vi "EventPassState.vi"(10 "IA State Input":T1) -> (1 "Id":dbl, 2 "IA State Output":T1, 3 "Pass State":bool)   [LabVIEW 2017]
uses:
  Core/AI Input.ctl
  Core/AI Robot.ctl
  Intel/Functions Enum.ctl
  Intel/AttackerStates.ctl
  Core/AI Ball.ctl
  Core/Field Size.ctl
  Core/AI Judge.ctl
  Intel/Command Enum.ctl
  Events.ctl
panel:
  in  "Desabilita passe":bool=TRUE
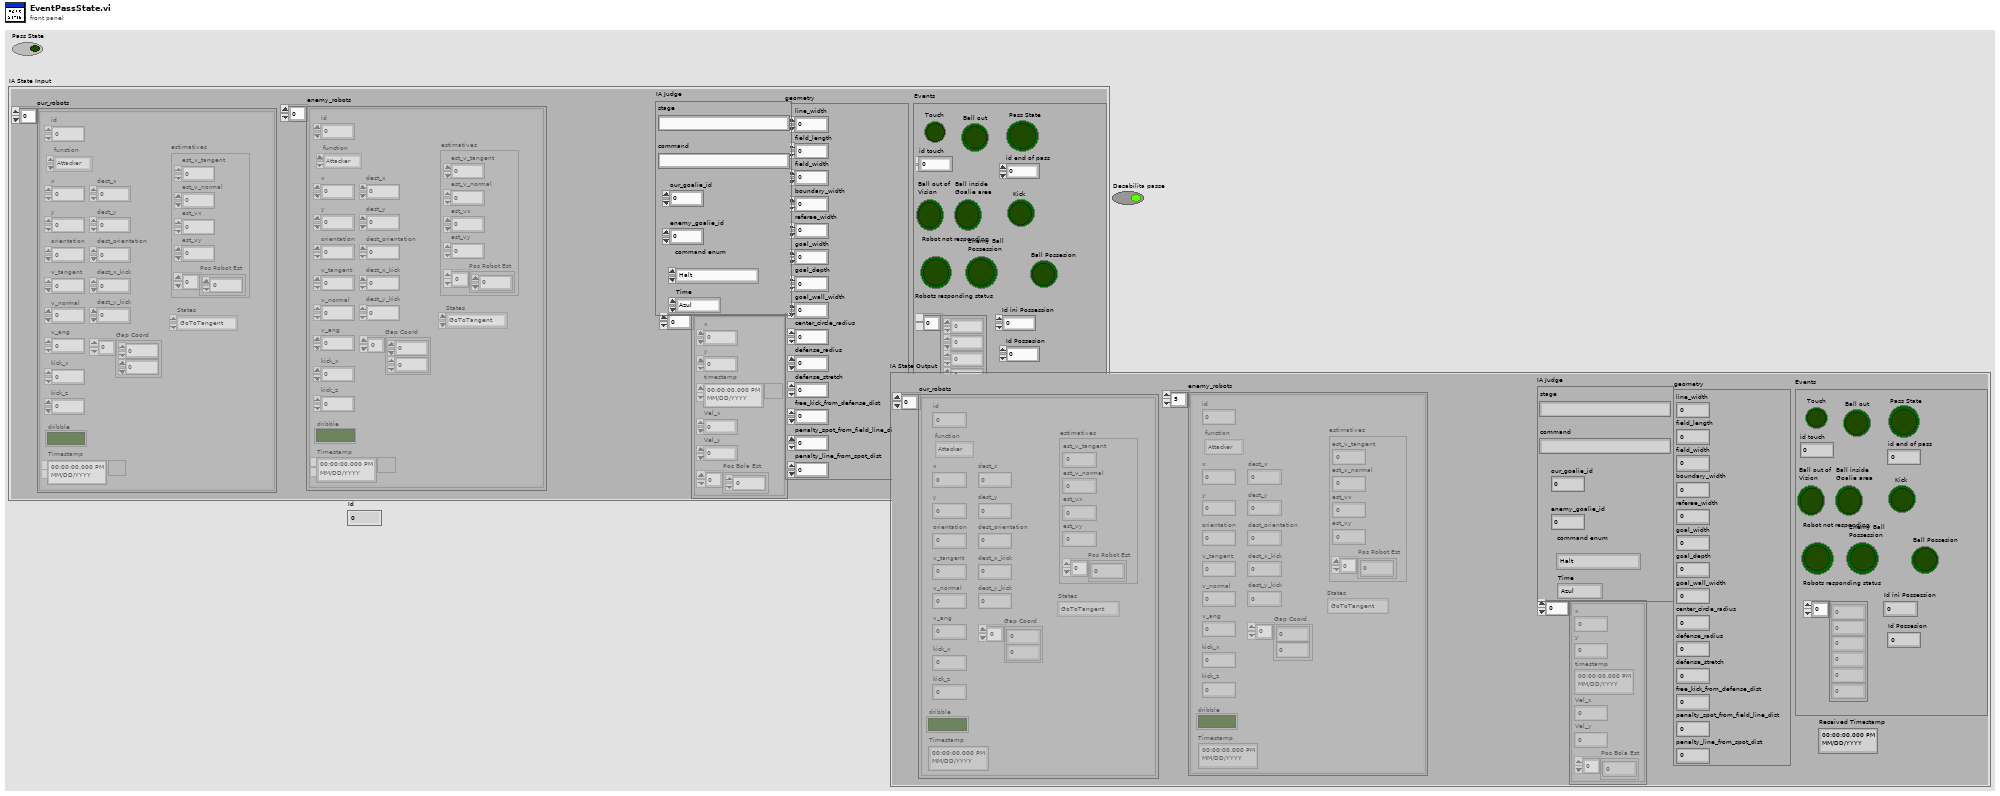
[diagram p1: front panel]
types:
  T1 = typedef "AI Input.ctl" = cluster{"our_robots":T2[], "enemy_robots":T2[], "balls":T5[], "geometry":T6, "IA Judge":T7, "Received Timestamp":timestamp, "Events":T9}
  T2 = typedef "AI Robot.ctl" = cluster{"id":u32, "function":T3, "x":dbl, "y":dbl, "orientation":dbl, "v_tangent":dbl, "v_normal":dbl, "v_ang":dbl, "kick_x":dbl, "kick_z":dbl, "dribble":bool, "Timestamp":timestamp, "dest_x":dbl, "dest_y":dbl, "dest_orientation":dbl, "estimatives":cluster{"est_v_tangent":dbl, "est_v_normal":dbl, "est_vx":dbl, "est_vy":dbl, "Pos Robot Est":dbl[]}, "dest_x_kick":dbl, "dest_y_kick":dbl, "Gap Coord":dbl[], "States":T4}
  T3 = typedef "Functions Enum.ctl" = enum16{"Attacker", "Goalie", "Defender", "Striker", "Goto 0", "Dummy", "Kicker", "ZigZag"}
  T4 = typedef "AttackerStates.ctl" = enum16{"Pass", "GoToTangent", "BallGetting", "GoToKick", ""}
  T5 = typedef "AI Ball.ctl" = cluster{"x":dbl, "y":dbl, "timestamp":timestamp, "Vel_x":dbl, "Vel_y":dbl, "Pos Bola Est":dbl[]}
  T6 = typedef "Field Size.ctl" = cluster{"line_width":u32, "field_length":u32, "field_width":u32, "boundary_width":u32, "referee_width":u32, "goal_width":u32, "goal_depth":u32, "goal_wall_width":u32, "center_circle_radius":u32, "defense_radius":u32, "defense_stretch":u32, "free_kick_from_defense_dist":u32, "penalty_spot_from_field_line_dist":u32, "penalty_line_from_spot_dist":u32}
  T7 = typedef "AI Judge.ctl" = cluster{"stage":string, "command":string, "our_goalie_id":dbl, "enemy_goalie_id":dbl, "command enum":T8, "Time":enum16{"Azul", "Amarelo"}}
  T8 = typedef "Command Enum.ctl" = enum16{"Halt", "Stop", "Force Start", "PKA Normal Start", "Prepare Kickoff Ally", "PKE Normal Start", "Prepare Kickoff Enemy", "Prepare Penalty Ally", "PPA Normal Start", "Prepare Penalty Enemy", "PPE Normal Start", "Direct Free Enemy", "Direct Free Ally", "Indirect Free Enemy", "Indirect Free Ally", "Timeout Enemy", "Timeout Ally", "Goal Enemy", "Goal Ally", "Ball Placement Enemy", "Ball Placement Ally", "Normal Half Time", "Extra Time Break", "Extra Half Time", "None", "Post Game"}
  T9 = typedef "Events.ctl" = cluster{"Touch":bool, "Ball out":bool, "id touch":dbl, "Ball out of \nVision":bool, "Ball inside \nGoalie area":bool, "Robot not responding":bool, "Robots responding status":dbl[], "Enemy Ball \nPossession":bool, "Pass State":bool, "id end of pass":dbl, "Kick":bool, "Id ini Possession":dbl, "Ball Possesion":bool, "Id Possesion":dbl}
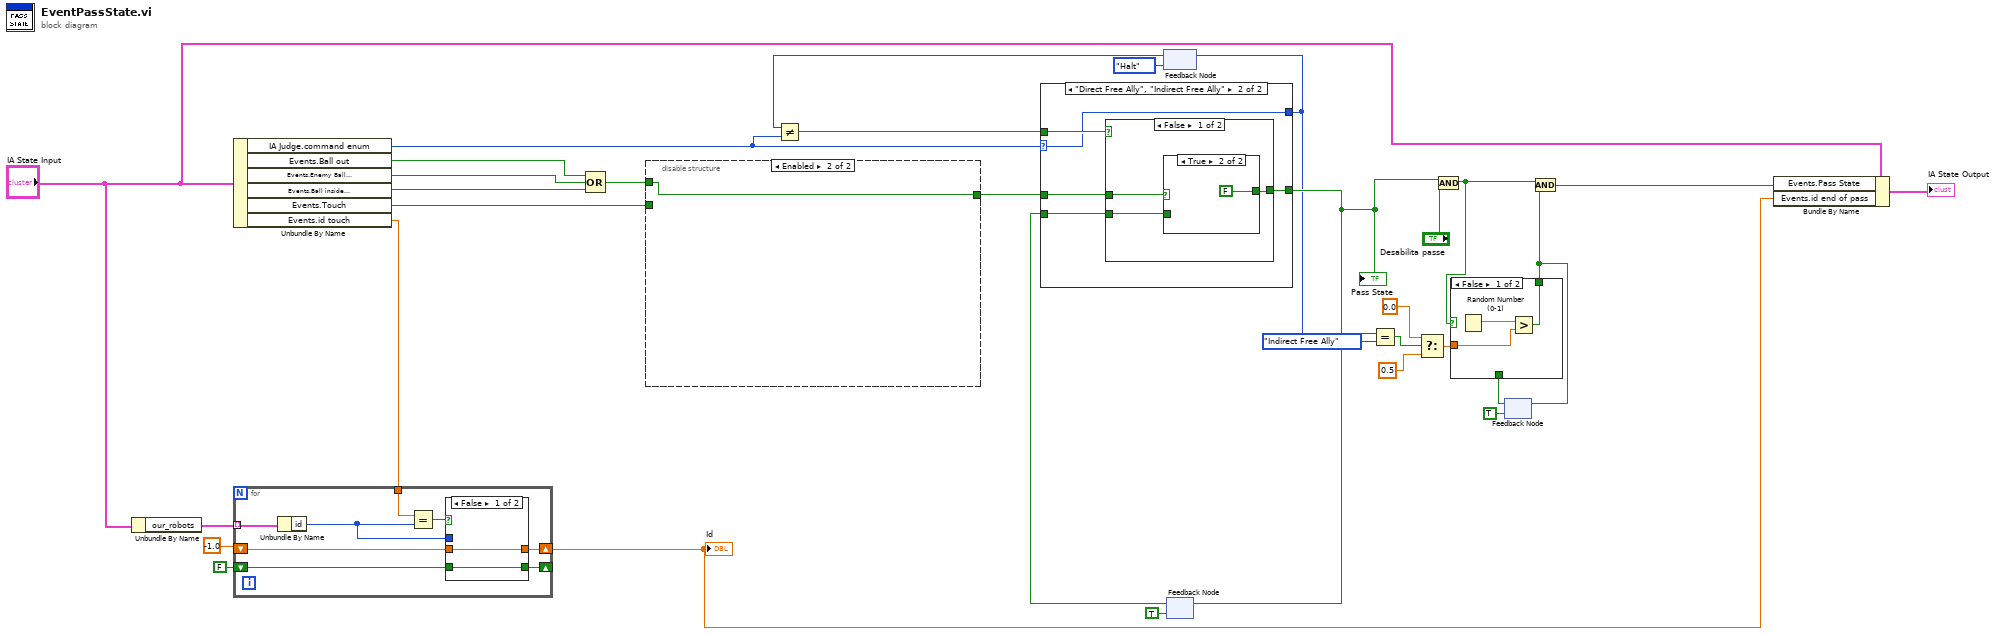
[diagram p0: block diagram]
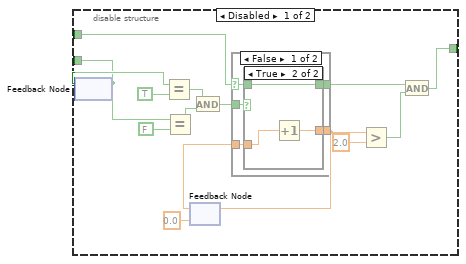
[diagram p3: hidden frame]
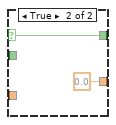
[diagram p5: hidden frame]
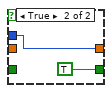
[diagram p6: hidden frame]
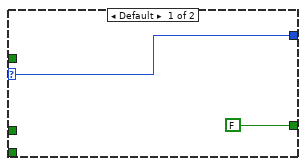
[diagram p7: hidden frame]
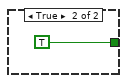
[diagram p9: hidden frame]
diagram:
  n1 = Unbundle By Name("IA State Input") -> ("our_robots"=w26:T2[])
  n2 = Unbundle By Name("IA State Input") -> ("IA Judge.command enum"=w32:T8, "Events.Ball out"=w18:bool, "Events.Enemy Ball \nPossession"=w17:bool, "Events.Ball inside \nGoalie area"=w16:bool, "Events.Touch"=w19:bool, "Events.id touch"=w25:dbl)
  n3 = for {
    tunnel: w26 -> [w40] mode=indexing
    shift-right: [w37] -> _
    shift-left: FALSE -> [w38]
    tunnel: w25 -> [w39]
    shift-right: [w34] -> w20
    shift-left: -1.0 -> [w33]
    n4 = Unbundle By Name(w40) -> ("id"=w35:u32)
    n5 = Equal?(x=w39, y=w35) -> (x = y?=w36:bool)
    n6 = case shown="False" w36 {
      tunnel: w38 -> [w42 _]
      tunnel: [w42 TRUE] -> w37
      tunnel: w35 -> [_ w43]
      tunnel: [w41 w43] -> w34
      tunnel: w33 -> [w41 _]
      frame False {
      }
      frame True {
      }
    }
  }
  "Id" <- w20
  n7 = Compound Arithmetic op=OR(w18, w17, w16) -> (w15:bool)
  n8 = disable-structure shown="Enabled" {
    disable-tunnel: w19 -> [w58 _]
    disable-tunnel: w15 -> [w48 w72]
    disable-tunnel: [w45 w72] -> w14
    frame Disabled {
      n9 = feedback #1() -> (w59:bool)  [unwired: 1 in]
      n10 = feedback-in #1(w58) -> ()
      n11 = Equal?(x=w59, y=TRUE) -> (x = y?=w55:bool)
      n12 = Equal?(x=w58, y=FALSE) -> (x = y?=w54:bool)
      n13 = feedback #2(0.0) -> (w52:dbl)
      n14 = And(x=w55, y=w54) -> (x .and. y?=w53:bool)
      n15 = case shown="False" w48 {
        selector: w48 -> [w61 w70]
        tunnel: w53 -> [w64 _]
        tunnel: w52 -> [w63 _]
        tunnel: [w62 0.0] -> w50
        tunnel: [w60 w70] -> w46
        frame False {
          n16 = case shown="True" w64 {
            tunnel: [w66 w69] -> w62
            tunnel: w63 -> [w66 w68]
            tunnel: w61 -> [w65 w67]
            tunnel: [w65 w67] -> w60
            frame False {
            }
            frame True {
              n17 = Increment(x=w68) -> (x+1=w69:dbl)
            }
          }
        }
        frame True {
        }
      }
      n18 = feedback-in #2(w50) -> ()
      n19 = Greater?(x=w50, y=2.0) -> (0:w47:bool)
      n20 = And(x=w46, y=w47) -> (x .and. y?=w45:bool)
    }
    frame Enabled {
    }
  }
  n21 = feedback #3(Command_Enum."Halt" ("command\nenum")) -> (w31:T8)
  n22 = Not Equal?(x=w31, y=w32) -> (x != y?=w30:bool)
  n23 = feedback #4(TRUE) -> (w29:bool)
  n24 = case shown="\"Direct Free Ally\", \"Indirect Free Ally\"" w32 {
    selector: w32 -> [w73 w75]
    tunnel: w14 -> [_ w79]
    tunnel: w30 -> [_ w78]
    tunnel: [FALSE w77] -> w13
    tunnel: w29 -> [_ w76]
    tunnel: [w73 w75] -> w6
    frame Default {
    }
    frame "Direct Free Ally", "Indirect Free Ally" {
      n25 = case shown="False" w78 {
        tunnel: w79 -> [w82 _]
        tunnel: [w81 TRUE] -> w77
        tunnel: w76 -> [w80 _]
        frame False {
          n26 = case shown="True" w82 {
            tunnel: [w83 FALSE] -> w81
            tunnel: w80 -> [w83 _]
            frame False {
            }
            frame True {
            }
          }
        }
        frame True {
        }
      }
    }
  }
  "Pass State" <- w13
  n27 = feedback-in #3(w6) -> ()
  n28 = feedback-in #4(w13) -> ()
  n29 = Equal?(x=w6, y=Command_Enum."Indirect Free Ally") -> (x = y?=w3:bool)
  n30 = Select(t=0.0, s=w3, f=0.5 ("y")) -> (s? t:f=w1:dbl)
  n31 = And(x=w13, y="Desabilita passe") -> (x .and. y?=w10:bool)
  n32 = feedback #5(TRUE) -> (w9:bool)
  n33 = case shown="False" w10 {
    tunnel: [w87 w89] -> w7
    tunnel: w9 -> [_ w89]
    tunnel: w1 -> [w86 _]
    frame False {
      n34 = Random Number (0-1)() -> (number: 0 to 1=w88:dbl)
      n35 = Greater?(x=w88, y=w86) -> (0:w87:bool)
    }
    frame True {
    }
  }
  n36 = feedback-in #5(w7) -> ()
  n37 = And(x=w10, y=w7) -> (x .and. y?=w11:bool)
  n38 = Bundle By Name(cluster="IA State Input", "Events.Pass State"=w11, "Events.id end of pass"=w20) -> (→"IA State Output":T1)
